vi "主界面main.vi"() -> ()   [LabVIEW 2023]
doc: "This VI illustrates how to create a sound file using microphone input as data. It displays the sound data in a graph as it is written to the file."
uses:
  <vilib>/sound2/lvsound2.llb/Sampling Mode.ctl
  <vilib>/sound2/lvsound2.llb/Sound Data Format.ctl
  global_variable.vi
  <vilib>/sound2/lvsound2.llb/Sound File Write Open.vi
  <vilib>/sound2/lvsound2.llb/Sound Input Read (DBL).vi
  <vilib>/sound2/lvsound2.llb/Sound File Write (DBL).vi
  <vilib>/Utility/file.llb/Read From Spreadsheet File (string).vi
panel:
  out "Boolean":bool
  out "String 2":string
  in  "退出系统":bool
  out "Generated Sound File":path
  in  "Device ID":u32
  in  "Tab Control":enum32{"出入门识别", "数据管理"}(tab)
  out "Waveform Graph":waveform(dbl)[](graph)
  in  "语音录入开始":bool
  in  "语音录入停止":bool
  out "String":string
  in  "信息查看":bool
  in  "信息采集":bool
  in  "身份":string(combo)
  in  "确定":bool
  in  "管理密码":string
  in  "进出记录":bool
  # "上海理工大学门禁系统"
  # "usst"
  # "语音录入时间"
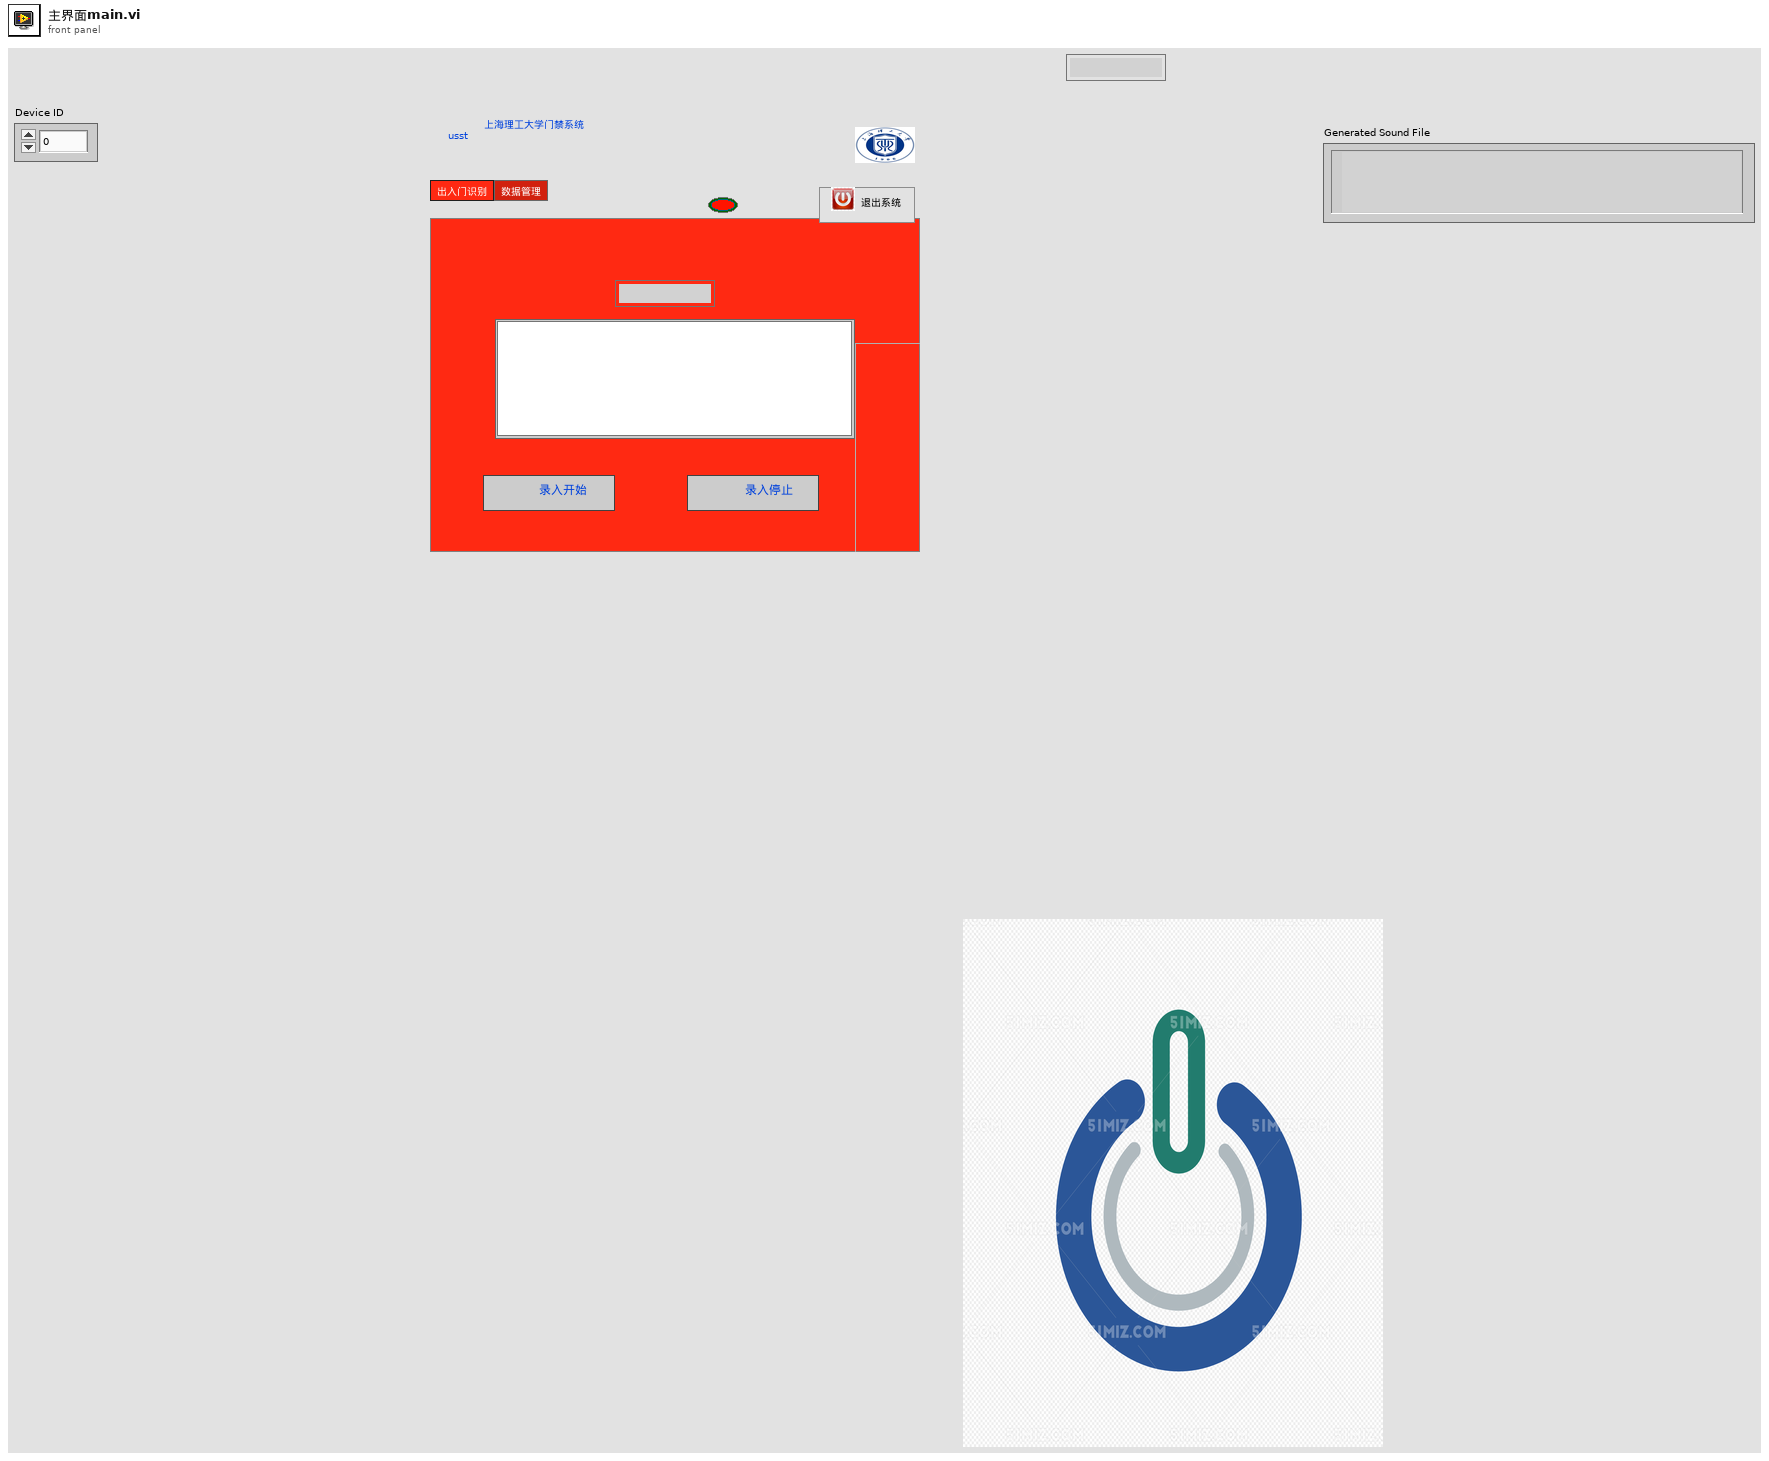
[diagram p1: front panel]
types:
  T1 = enum8{"Enabled", "Disabled", "Disabled and Grayed Out"}
  T2 = typedef "Sound Data Format.ctl" = cluster{"sample rate (S/s)":dbl, "number of channels":i32, "bits per sample":i32}
  T3 = typedef "Sampling Mode.ctl" = i32
  T4 = typedef "Sound File Refnum.ctl" = refnum<file>
  T5 = typedef "Sound Input Task ID.ctl" = u32
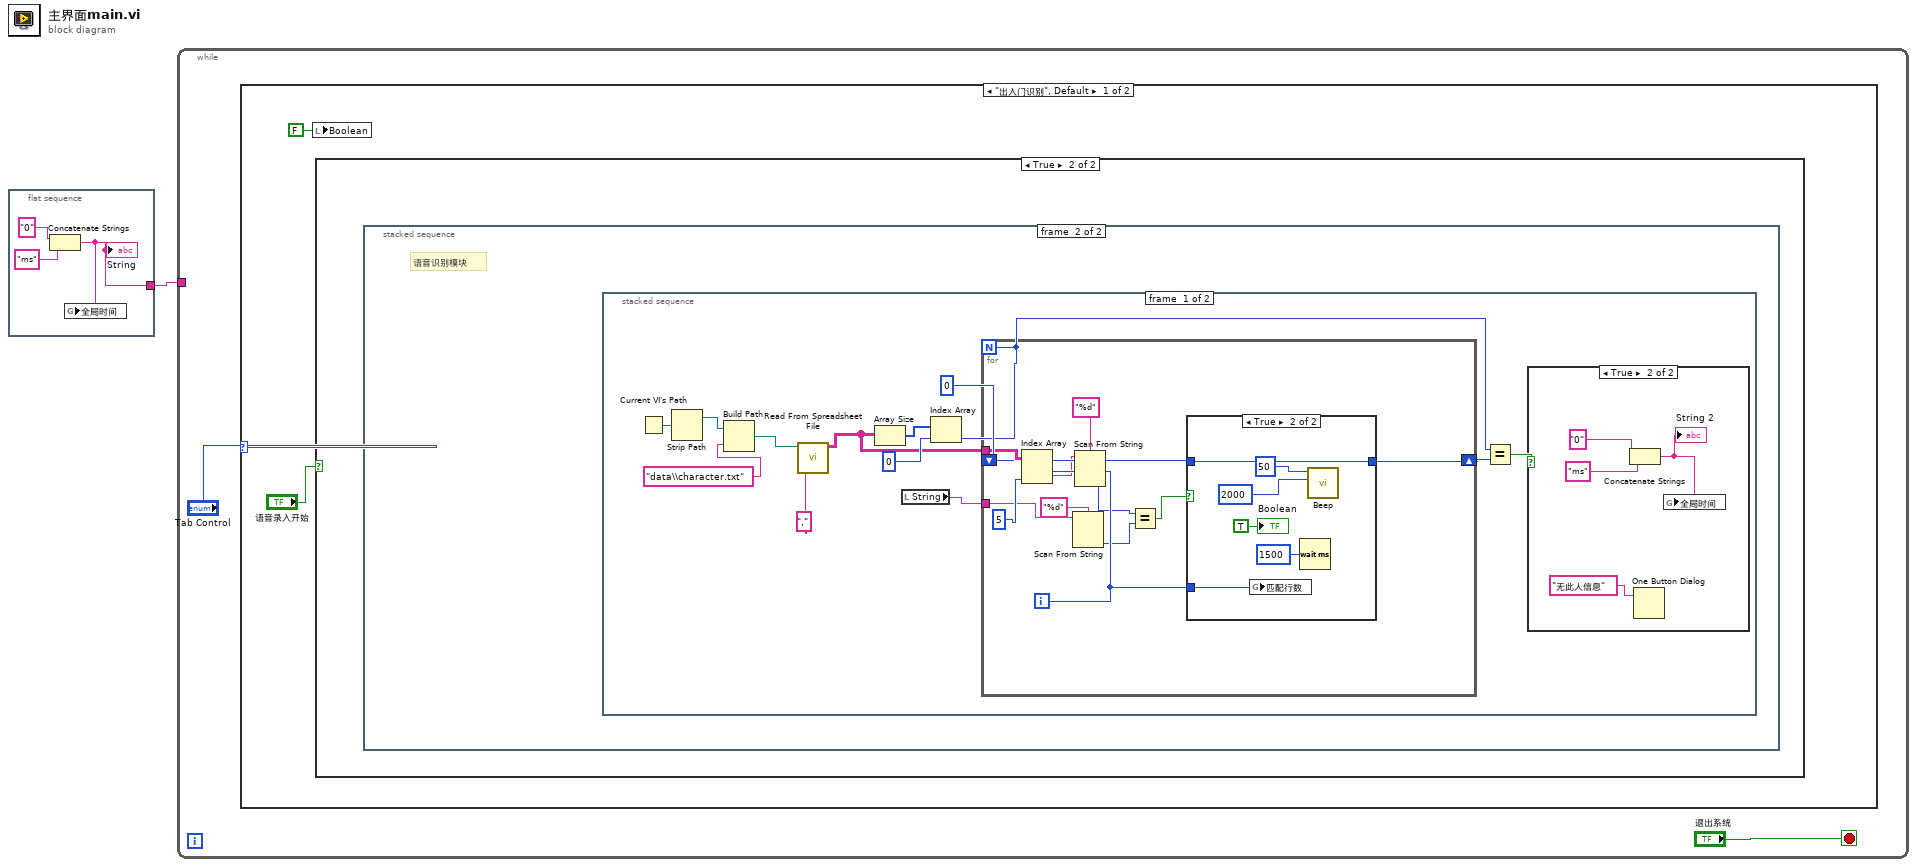
[diagram p0: block diagram]
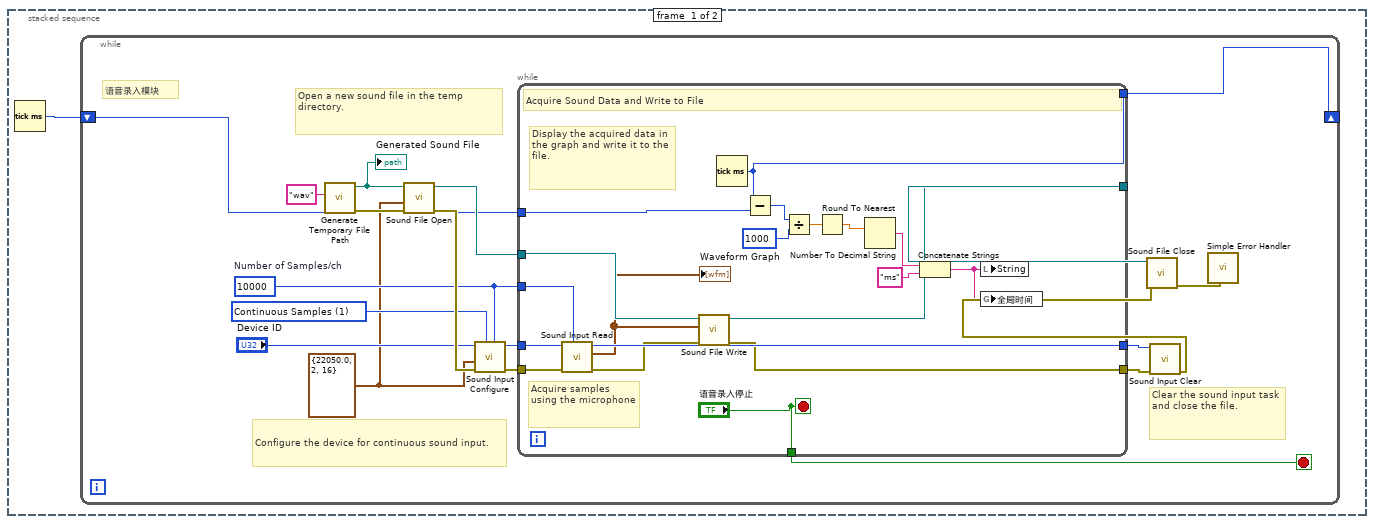
[diagram p3: hidden frame]
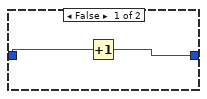
[diagram p5: hidden frame]
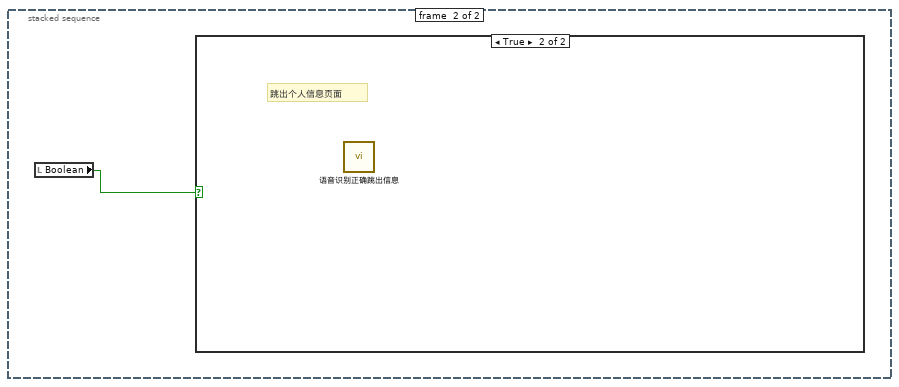
[diagram p6: hidden frame]
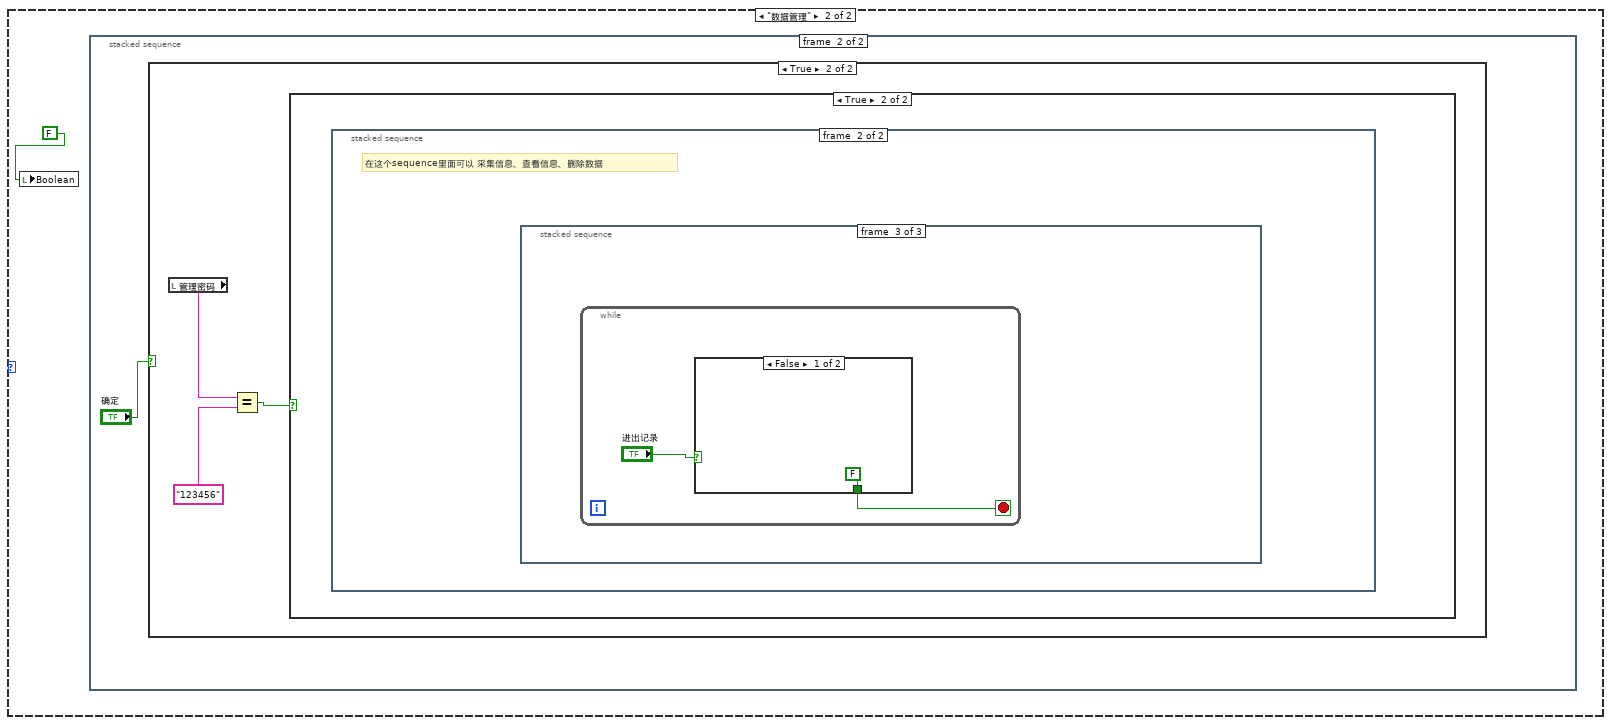
[diagram p8: hidden frame]
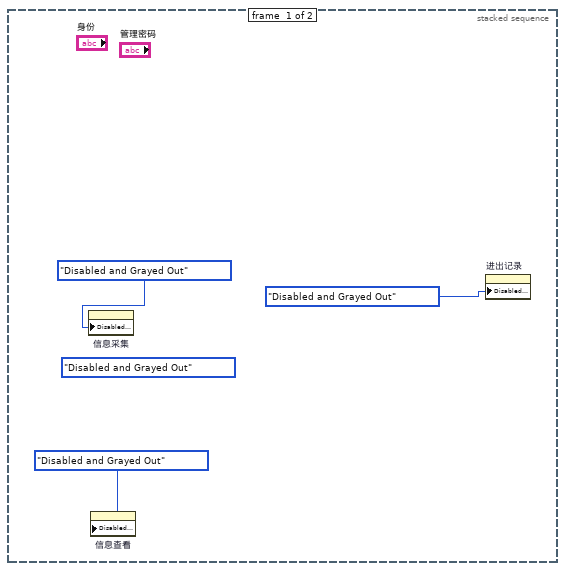
[diagram p9: hidden frame]
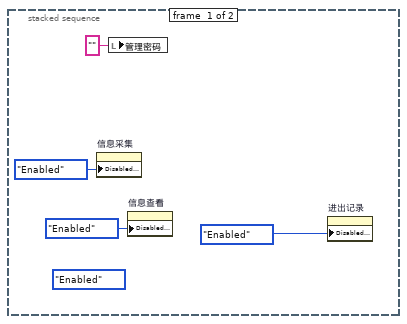
[diagram p12: hidden frame]
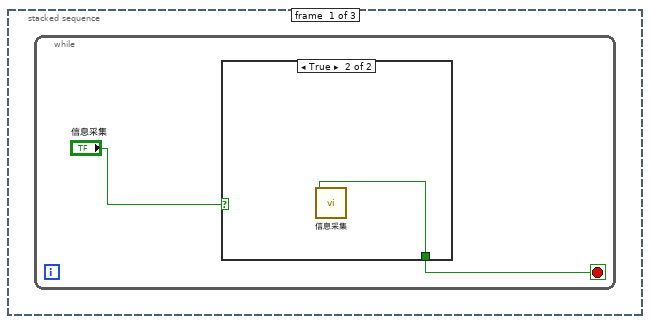
[diagram p13: hidden frame]
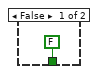
[diagram p14: hidden frame]
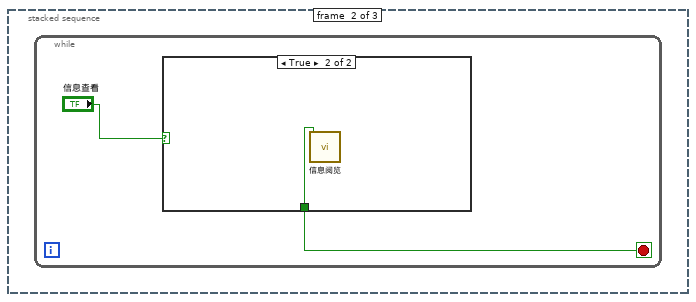
[diagram p15: hidden frame]
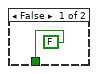
[diagram p16: hidden frame]
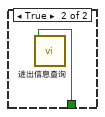
[diagram p17: hidden frame]
diagram:
  n1 = flat-sequence {
    tunnel: [w2] -> w1
    frame #0 {
      n2 = Concatenate Strings("0" ("string"), "ms" ("string")) -> (w2:string)
      "String" <- w2
      n3 = global write "global_variable.vi" "全局时间"(w2) -> ()
    }
  }
  n4 = while {
    tunnel: w1 -> [_]
    stop <- "退出系统" stop-if-true
    n5 = case shown="\"出入门识别\", Default" "Tab Control" {
      frame "出入门识别", Default {
        n6 = local write "Boolean"(FALSE ("Boolean")) -> ()
        n7 = case shown="True" "语音录入开始" {
          frame False {
          }
          frame True {
            n8 = stacked-sequence {
              frame #0 {
                n9 = Tick Count (ms)() -> (millisecond timer value=w9:u32)
                n10 = while {
                  shift-right: [w11] -> _
                  shift-left: w9 -> [w10]
                  stop <- w12 stop-if-true
                  w14 = T2 {"sample rate (S/s)"=22050.0, "number of channels"=2, "bits per sample"=16} ("Sound Format")
                  w16 = 10000  # Number of Samples/ch
                  w15 = T3 1 items=["Finite Samples", "Continuous Samples"] ("sample mode")
                  # "语音录入模块"
                  # "Configure the device for continuous sound input."
                  # "Clear the sound input task and close the file."
                  # "Open a new sound file in the temp directory."
                  n11 = call <vilib>:"Generate Temporary File Path.vi"("Temporary File Extension (tmp)"="wav") -> ("error out"=w27:errorcluster, "Unique Temporary File Path"=w28:path)  [unwired: 9 in]
                  "Generated Sound File" <- w28
                  n12 = call-poly <vilib>:"Sound File Open.vi"("error in (no error)"=w27, "sound format"=w14, "path"=w28) -> ("error out"=w25:errorcluster, "sound file refnum"=w22:T4)  [unwired: 7 in]
                  n13 = call <vilib>:"Sound Input Configure.vi"("number of samples/ch"=w16, "sample mode"=w15, "error in (no error)"=w25, "sound format"=w14, "device ID"="Device ID") -> ("error out"=w17:errorcluster, "task ID"=w19:T5)  [unwired: 5 in]
                  n14 = while {
                    tunnel: w16 -> [w44]
                    tunnel: w22 -> [w43]
                    tunnel: [w42] -> w23
                    tunnel: w19 -> [w46]
                    tunnel: [w45] -> w20
                    tunnel: w17 -> [w47]
                    tunnel: [w39] -> w21
                    tunnel: ["语音录入停止"] -> w12
                    tunnel: [w37] -> w11
                    tunnel: w10 -> [w36]
                    stop <- "语音录入停止" stop-if-true
                    # "Acquire samples using the microphone"
                    # "Display the acquired data in the graph and write it to the file."
                    # "Acquire Sound Data and Write to File"
                    n15 = call-poly <vilib>:"Sound Input Read.vi"("number of samples/ch"=w44, "error in (no error)"=w47, "task ID"=w46) -> ("error out"=w41:errorcluster, "data"=w40:waveform(dbl)[], "task ID out"=w45:T5)  [unwired: 6 in]
                    "Waveform Graph" <- w40
                    n16 = call-poly <vilib>:"Sound File Write.vi"("error in (no error)"=w41, "data"=w40, "sound file refnum"=w43) -> ("error out"=w39:errorcluster, "sound file refnum out"=w42:T4)  [unwired: 7 in]
                    n17 = Tick Count (ms)() -> (millisecond timer value=w37:u32)
                    n18 = Subtract(x=w37, y=w36) -> (x-y=w34:u32)
                    n19 = Divide(x=w34, y=u32 1000) -> (x/y=w31:dbl)
                    n20 = Round To Nearest(number=w31) -> (nearest integer value=w30:dbl)
                    n21 = Number To Decimal String(number=w30) -> (decimal integer string=w33:string)  [unwired: 1 in]
                    n22 = Concatenate Strings(w33, "ms" ("string")) -> (w29:string)
                    n23 = local write "String"(w29) -> ()
                    n24 = global write "global_variable.vi" "全局时间"(w29) -> ()
                  }
                  n25 = call <vilib>:"Sound Input Clear.vi"("error in (no error)"=w21, "task ID"=w20) -> ("error out"=w24:errorcluster)  [unwired: 9 in]
                  n26 = call <vilib>:"Sound File Close.vi"("error in (no error)"=w24, "sound file refnum"=w23) -> ("error out"=w26:errorcluster)  [unwired: 9 in]
                  n27 = call <vilib>:"Simple Error Handler.vi"("error in (no error)"=w26) -> ()  [unwired: 4 in, 5 out]
                }
              }
              frame #1 {
                # "语音识别模块"
                n28 = stacked-sequence {
                  frame #0 {
                    n29 = Current VI's Path() -> (path=w60:path)
                    n30 = Strip Path(path=w60) -> (stripped path=w59:path)  [unwired: 1 out]
                    n31 = Build Path(base path=w59, name or relative path="data\\character.txt") -> (appended path=w53:path)
                    n32 = call-poly <vilib>:"Read From Spreadsheet File.vi"("delimiter (\\t)"=",", "file path (dialog if empty)"=w53) -> ("all rows"=w54:string[][])  [unwired: 5 in, 4 out]
                    n33 = Array Size(array=w54) -> (size(s)=w56:i32[])
                    n34 = local read "String"() -> (w52:string)
                    n35 = Index Array(array=w56, index=0 ("index (row)")) -> (element=w50:i32)
                    n36 = for {
                      N: w50 -> [_]
                      tunnel: w54 -> [w76]
                      tunnel: w52 -> [w67]
                      shift-right: [w72] -> w49
                      shift-left: 0 -> [w73]
                      i -> [w71]
                      n37 = Index Array(array=w76, index (row)=w71, index (col)=5 ("disabled index (col)")) -> (element=w70:string)
                      n38 = Scan From String(format string="%d", input string=w67) -> (output 1=w66:i32)  [unwired: 3 in, 3 out]
                      n39 = Scan From String(format string="%d", input string=w70) -> (output 1=w65:i32)  [unwired: 3 in, 3 out]
                      n40 = Equal?(x=w65, y=w66) -> (x = y?=w74:bool)
                      n41 = case shown="True" w74 {
                        tunnel: w73 -> [w78 w84]
                        tunnel: [w77 w84] -> w72
                        tunnel: w71 -> [_ w83]
                        frame False {
                          n42 = Increment(x=w78) -> (x+1=w77:i32)
                        }
                        frame True {
                          n43 = global write "global_variable.vi" "匹配行数"(w83) -> ()
                          n44 = Wait (ms)(milliseconds to wait=u32 1500) -> ()  [unwired: 1 out]
                          n45 = call <vilib>:"Beep.vi"("duration (msec)"=u32 2000, "frequency (Hz)"=u32 50) -> ()  [unwired: 10 in]
                          "Boolean" <- TRUE ("Boolean")
                        }
                      }
                    }
                    n46 = Equal?(x=w50, y=w49) -> (x = y?=w48:bool)
                    n47 = case shown="True" w48 {
                      frame False {
                      }
                      frame True {
                        n48 = Concatenate Strings("0" ("string"), "ms" ("string")) -> (w63:string)
                        "String 2" <- w63
                        n49 = One Button Dialog(message="无此人信息") -> ()  [unwired: 1 in, 1 out]
                        n50 = global write "global_variable.vi" "全局时间"(w63) -> ()
                      }
                    }
                  }
                  frame #1 {
                    n51 = local read "Boolean"() -> (w85:bool)
                    n52 = case shown="True" w85 {
                      frame False {
                      }
                      frame True {
                        # "跳出个人信息页面"
                        n53 = call "语音识别正确跳出信息.vi"() -> ()  [unwired: 10 in, 1 out]
                      }
                    }
                  }
                }
              }
            }
          }
        }
      }
      frame "数据管理" {
        n54 = local write "Boolean"(FALSE ("Boolean")) -> ()
        n55 = stacked-sequence {
          frame #0 {
            (unwired) T1."Disabled and Grayed Out" ("Disabled")
            n56 = property on="信息采集" class="Bool"("DisabledEnum"=T1."Disabled and Grayed Out" ("Disabled")) -> ()  [unwired: 2 in, 2 out]
            n57 = property on="信息查看" class="Bool"("DisabledEnum"=T1."Disabled and Grayed Out" ("Disabled")) -> ()  [unwired: 2 in, 2 out]
            n58 = property on="进出记录" class="Bool"("DisabledEnum"=T1."Disabled and Grayed Out" ("Disabled")) -> ()  [unwired: 2 in, 2 out]
          }
          frame #1 {
            n59 = case shown="True" "确定" {
              frame False {
              }
              frame True {
                n60 = local read "管理密码"() -> (w93:string)
                n61 = Equal?(x=w93, y="123456") -> (x = y?=w91:bool)
                n62 = case shown="True" w91 {
                  frame False {
                  }
                  frame True {
                    n63 = stacked-sequence {
                      frame #0 {
                        (unwired) T1."Enabled" ("Disabled")
                        n64 = property on="信息采集" class="Bool"("DisabledEnum"=T1."Enabled" ("Disabled")) -> ()  [unwired: 2 in, 2 out]
                        n65 = local write "管理密码"("" ("管理密码")) -> ()
                        n66 = property on="信息查看" class="Bool"("DisabledEnum"=T1."Enabled" ("Disabled")) -> ()  [unwired: 2 in, 2 out]
                        n67 = property on="进出记录" class="Bool"("DisabledEnum"=T1."Enabled" ("Disabled")) -> ()  [unwired: 2 in, 2 out]
                      }
                      frame #1 {
                        # "在这个sequence里面可以 采集信息、查看信息、删除数据"
                        n68 = stacked-sequence {
                          frame #0 {
                            n69 = while {
                              stop <- w98 stop-if-true
                              n70 = case shown="True" "信息采集" {
                                tunnel: [FALSE ("Boolean") w101] -> w98
                                frame False {
                                }
                                frame True {
                                n71 = call "信息采集.vi"() -> ("Boolean"=w101:bool)  [unwired: 11 in]
                                }
                              }
                            }
                          }
                          frame #1 {
                            n72 = while {
                              stop <- w102 stop-if-true
                              n73 = case shown="True" "信息查看" {
                                tunnel: [FALSE ("信息查看完毕") w105] -> w102
                                frame False {
                                }
                                frame True {
                                n74 = call "信息阅览.vi"() -> ("输出完毕"=w105:bool)  [unwired: 11 in]
                                }
                              }
                            }
                          }
                          frame #2 {
                            n75 = while {
                              stop <- w106 stop-if-true
                              n76 = case shown="False" "进出记录" {
                                tunnel: [FALSE ("Boolean") w109] -> w106
                                frame False {
                                }
                                frame True {
                                n77 = call "进出信息查询.vi"() -> ("Boolean"=w109:bool)  [unwired: 11 in]
                                }
                              }
                            }
                          }
                        }
                      }
                    }
                  }
                }
              }
            }
          }
        }
      }
    }
  }
